vi "UHR-Fleezers Control (host) - 12.1_Jonathan.vi"() -> ()   [LabVIEW 2012] (continued)
                n283 = local read "Scan lines (y)"() -> (w520:u64)
                n284 = disable-structure shown="Disabled" {
                  frame Disabled {
                  }
                  frame Enabled {
                  }
                }
                n285 = local read "Actual MCL Inc (V)"() -> (w514:dbl)
                n286 = local read "Scan steps (MCL)"() -> (w519:u64)
                n287 = Divide "Y Pix/step"(x=w515, y=w520) -> (x/y=w527:dbl)
                n288 = Divide "Y V/pix"(x=w514, y=w527) -> (x/y=w526:dbl)
                n289 = Divide "Y half step offset"(x=w514, y=2.0) -> (x/y=w528:dbl)
                n290 = Divide "X pix/step"(x=w516, y=w519) -> (x/y=w525:dbl)
                n291 = Negate(x=w528) -> (-x=w529:dbl)
                n292 = local read "Initial Y"() -> (w535:dbl)
                n293 = Multiply(x=w517, y=w526) -> (x*y=w536:dbl)
                n294 = Divide "X half step offset"(x=w514, y=2.0) -> (x/y=w522:dbl)
                n295 = Divide "X V/pix"(x=w514, y=w525) -> (x/y=w524:dbl)
                n296 = Multiply(x=w514, y=w519) -> (x*y=w531:dbl)
                n297 = Compound Arithmetic op=ADD(w529, w536, w535) -> (w506:dbl)
                "Pointer Y (V)" <- w506
                n298 = Multiply(x=w524, y=w518) -> (x*y=w533:dbl)
                n299 = Negate(x=w522) -> (-x=w521:dbl)
                n300 = local read "Initial X"() -> (w534:dbl)
                n301 = Negate(x=w533) -> (-x=w532:dbl)
                n302 = Compound Arithmetic op=ADD(w521, w531, w534, w532) -> (w507:dbl)
                "Pointer X (V)" <- w507
                n303 = case shown="True" "Set High F Confocal Spot (X-Y)" {
                  tunnel: w507 -> [_ w537]
                  tunnel: w506 -> [_ w538]
                  frame False {
                  }
                  frame True {
                    "Confocal Y 2 (V)" <- w538
                    "Confocal X 2 (V)" <- w537
                  }
                }
                n304 = Or(x="Set X Only", y="Set Confocal Spot (X-Y)") -> (x .or. y?=w510:bool)
                n305 = Or(x="Set Confocal Spot (X-Y)", y="Set Y Only") -> (x .or. y?=w509:bool)
                n306 = case shown="True" w510 {
                  tunnel: w507 -> [_ w539]
                  frame False {
                  }
                  frame True {
                    n307 = property on="AO2" class="Slide (strict)"("Val(Sgnl)"=w539) -> ()  [unwired: 2 in, 2 out]
                    "Confocal X 1 (V)" <- w539
                  }
                }
                n308 = case shown="True" w509 {
                  tunnel: w506 -> [_ w540]
                  frame False {
                  }
                  frame True {
                    n309 = property on="AO1" class="Slide (strict)"("Val(Sgnl)"=w540) -> ()  [unwired: 2 in, 2 out]
                    "Confocal Y 1 (V)" <- w540
                  }
                }
                n310 = local write "Set High F Confocal Spot (X-Y)"(w505) -> ()
                n311 = local write "Set Confocal Spot (X-Y)"(w505) -> ()
                n312 = local write "Set X Only"(w505) -> ()
                n313 = local write "Set Y Only"(w505) -> ()
              }
            }
          }
          frame 3 {
            n314 = local read "BD 2 Frequency 1 (MHz)"() -> (w541:dbl)
            n315 = local read "BD 1 Frequency 1 (MHz)"() -> (w542:dbl)
            n316 = local write "Manipulating Trap"(TRUE ("Manipulating Trap")) -> ()
            n317 = local write "Coords"(T8 {"Horizontal"=0, "Vertical"=0} ("Coords")) -> ()
            n318 = while {
              tunnel: w547 -> [w552]
              tunnel: w545 -> [w551]
              tunnel: w543 -> [w550]
              tunnel: w542 -> [w549]
              tunnel: w541 -> [w548]
              stop <- w553 stop-if-true
              n319 = event shown="[0] \"Pane\": Mouse Move" {
                selector: _ -> [_ _]
                dyn-events: _ -> [_ _]
                timeout: _ -> [_ _]
                tunnel: ["Force Manip Abort" w617] -> w553
                tunnel: w552 -> [w560 _]
                tunnel: w551 -> [w558 _]
                tunnel: w550 -> [w557 _]
                tunnel: w549 -> [w556 _]
                tunnel: w548 -> [w555 _]
                event Mouse Move {
                  n320 = event-data() -> ("Time"=w561:u32, "Coords"=w562:T8)  [unwired: 3 out]
                  n321 = Less?(x=w561, y=w560) -> (x < y?=w559:bool)
                  n322 = case "Makes sure old motion events prior to mouse click aren't used" shown="False" w559 {
                    tunnel: w562 -> [w604 _]
                    tunnel: w558 -> [w605 _]
                    tunnel: w557 -> [w582 _]
                    tunnel: w556 -> [w578 _]
                    tunnel: w555 -> [w577 _]
                    frame False {
                      n323 = Subtract(x=w604, y=w605) -> (x-y=w603:T8)
                      "Coords" <- w603
                      n324 = local read "Y RF Frequency Limits (MHz)"() -> (w563:T17)
                      n325 = To Double Precision Float(number=w603) -> (double precision float=w602:cluster{"Horizontal":dbl, "Vertical":dbl})
                      n326 = Multiply(x=cluster{"Horizontal":dbl, "Vertical":dbl} {"Horizontal"=-1.0, "Vertical"=1.0}, y="Manipulation Scaling") -> (x*y=w598:cluster{"Horizontal":dbl, "Vertical":dbl})
                      n327 = local read "X RF Frequency Limits (MHz)"() -> (w564:T17)
                      n328 = Multiply(x=w602, y=w598) -> (x*y=w600:cluster{"Horizontal":dbl, "Vertical":dbl})
                      n329 = Unbundle By Name(w600) -> ("Horizontal"=w595:dbl, "Vertical"=w599:dbl)
                      n330 = Unbundle By Name(w563) -> ("Maximum"=w566:dbl, "Minimum"=w565:dbl)
                      n331 = Boolean To (0,1)(Boolean="Manip. X?") -> (0, 1=w593:i16)
                      n332 = Boolean To (0,1)(Boolean="Manip. Y?") -> (0, 1=w590:i16)
                      n333 = local read "BD 1 Frequency 2 (MHz)"() -> (w580:dbl)
                      n334 = Multiply(x=w599, y=w590) -> (x*y=w592:dbl)
                      n335 = Multiply(x=w593, y=w595) -> (x*y=w596:dbl)
                      n336 = local read "BD 2 Frequency 2 (MHz)"() -> (w579:dbl)
                      n337 = Unbundle By Name(w564) -> ("Maximum"=w568:dbl, "Minimum"=w567:dbl)
                      n338 = Add(x=w577, y=w592) -> (x+y=w570:dbl)
                      n339 = Add(x=w578, y=w596) -> (x+y=w572:dbl)
                      n340 = In Range and Coerce(upper limit=w568, x=w572, lower limit=w567) -> (coerced(x)=w571:dbl)  [unwired: 1 out]
                      n341 = In Range and Coerce(upper limit=w566, x=w570, lower limit=w565) -> (coerced(x)=w569:dbl)  [unwired: 1 out]
                      n342 = Subtract(x=w571, y=w580) -> (x-y=w589:dbl)
                      n343 = Subtract(x=w569, y=w579) -> (x-y=w588:dbl)
                      n344 = Square(x=w589) -> (x^2=w587:dbl)
                      n345 = Square(x=w588) -> (x^2=w586:dbl)
                      n346 = Add(x=w587, y=w586) -> (x+y=w585:dbl)
                      n347 = Square Root(x=w585) -> (sqrt(x)=w581:dbl)
                      n348 = In Range and Coerce(upper limit="Limit Max (MHz)", x=w581, lower limit="Limit Min (MHz)") -> (In Range?=w574:bool)  [unwired: 1 out]
                      n349 = Not(x="Limits Enable") -> (.not. x?=w573:bool)
                      n350 = Or(x=w574, y=w573) -> (x .or. y?=w575:bool)
                      n351 = case shown="True" w575 {
                        tunnel: w582 -> [_ w615]
                        tunnel: w581 -> [_ w606]
                        tunnel: w571 -> [_ w613]
                        tunnel: w580 -> [_ w612]
                        tunnel: w569 -> [_ w611]
                        tunnel: w579 -> [_ w610]
                        tunnel: w564 -> [_ w608]
                        tunnel: w563 -> [_ w607]
                        frame False {
                        }
                        frame True {
                          n352 = local read "BD 1 Frequency 3 (MHz)"() -> (w614:dbl)
                          n353 = local read "BD 2 Frequency 3 (MHz)"() -> (w609:dbl)
                          n354 = local write "Trap Delta (MHz)"(w606) -> ()
                          n355 = call "set RF board frequency - interlace.vi"("Board 2 Frequency Limits"=w607, "Board 1 Frequency Limits"=w608, "FPGA VI Reference In"=w615, "Board 2 Frequency 3 (MHz)"=w609, "Board 1 Frequency 3 (MHz)"=w614, "Board 2 Frequency 2 (MHz)"=w610, "Board 2 Frequency 1 (MHz)"=w611, "Board 1 Frequency 2 (MHz)"=w612, "Board 1 Frequency 1  (MHz)"=w613) -> ()  [unwired: 1 in, 2 out]
                          n356 = local write "BD 2 Frequency 1 (MHz)"(w611) -> ()
                          n357 = local write "BD 1 Frequency 1 (MHz)"(w613) -> ()
                        }
                      }
                    }
                    frame True {
                    }
                  }
                }
                event Mouse Up {
                  n358 = event-data() -> ("Button"=w616:u16)  [unwired: 8 out]
                  n359 = case shown="3" w616 {
                    tunnel: [FALSE TRUE] -> w617
                    frame 0, Default {
                    }
                    frame 3 {
                      n360 = local read "Trap Delta (MHz)"() -> (w619:dbl)
                      n361 = property on="Initial delta (MHz)" class="DigNum (strict)"("Val(Sgnl)"=w619) -> ()  [unwired: 2 in, 2 out]
                      n362 = local write "Manipulating Trap"(FALSE ("Manipulating Trap")) -> ()
                    }
                  }
                }
              }
            }
          }
        }
      }
      event Mouse Move {
        n363 = event-data() -> ()  [unwired: 6 out]
      }
    }
    n364 = local read "Stop All"() -> (w435:bool)
    n365 = node-c288() -> ()  [unwired: 2 out]
  }
  n366 = timed-loop "Run Scripts, including: stage motion" {
    tunnel: w91 -> [w628]
    tunnel: w90 -> [w629]
    tunnel: [w629] -> w89
    tunnel: [w628] -> w88
    timing: w86 -> [_]
    timing-out: [_] -> w85
    tunnel: w71 -> [w627]
    tunnel: w72 -> [w626]
    tunnel: w12 -> [w623]
    tunnel: w11 -> [w622]
    tunnel: w10 -> [w624]
    tunnel: w9 -> [w625]
    stop <- w630 stop-if-true
    n367 = node-c288() -> ()  [unwired: 1 in, 1 out]
    n368 = event shown="[3] \"Move Cap. 2 (ADig Top)\": Value Change" {
      selector: _ -> [_ _ _ _ _ _ _ _ _ _ _ _ _ _ _ _ _ _ _]
      dyn-events: _ -> [_ _ _ _ _ _ _ _ _ _ _ _ _ _ _ _ _ _ _]
      timeout: _ -> [_ _ _ _ _ _ _ _ _ _ _ _ _ _ _ _ _ _ _]
      tunnel: ["Set Position" "Move to Position" _ _ "Read Harvard" _ _ _ _ _ _ "Got ADig bead" "Force FB Data\nScript" _ "Got DNA bead" "Take Stepping Data" _ "Take Detection Laser\nImage" _] -> _
      tunnel: [_ _ _ _ _ _ _ _ _ _ _ _ _ _ _ _ _ _ w1247] -> w630
      tunnel: w628 -> [w648 w656 w669 w699 _ w744 w784 w865 w894 w1026 w1052 _ w1088 _ _ _ _ _ _]
      tunnel: w629 -> [w649 w657 w670 w700 _ w745 w785 w866 w895 w1027 w1053 _ w1089 _ _ _ _ _ _]
      tunnel: w627 -> [_ _ _ _ w729 _ _ _ _ _ _ _ _ _ _ _ _ _ _]
      tunnel: w626 -> [_ _ _ _ w728 _ _ _ _ _ _ _ _ _ _ _ _ _ _]
      tunnel: w625 -> [_ _ _ _ _ _ _ _ _ _ _ _ _ _ _ _ _ _ _]
      tunnel: w624 -> [_ _ _ _ _ _ _ _ _ _ _ _ _ _ _ _ _ _ _]
      tunnel: w623 -> [_ _ _ _ _ _ _ _ _ _ _ _ _ _ _ _ _ _ _]
      tunnel: w622 -> [_ _ _ _ _ _ _ _ _ _ _ _ _ _ _ _ _ _ _]
      event "Set Position", "Set Position 2", "Set Position 3", "Set Position 4", "Set Position 5", "Set Position 1": Value Change {
        n369 = event-data() -> ()  [unwired: 1 in, 5 out]
        n370 = Build Array("Set Position 1", "Set Position 2", "Set Position 3", "Set Position 4", "Set Position 5") -> (w647:bool[])
        n371 = Boolean Array To Number(Boolean array=w647) -> (number=w646:u32)
        n372 = Logarithm Base 2(1:w646) -> (0:w638:dbl)
        n373 = call "Read Stage Position.vi"("error in"=w648, "VISA resource name in"=w649) -> ("Current Position"=w653:cluster{dbl, dbl, dbl}, "error out"=w652:errorcluster)  [unwired: 2 out]
        n374 = Decrement(x="Position") -> (x-1=w636:dbl)
        n375 = Greater Or Equal?(x=w638, y=0.0) -> (x >= y?=w639:bool)
        n376 = Cluster To Array(cluster=w653) -> (array=w650:dbl[])
        n377 = local write "Stage Control Serial Error"(w652) -> ()
        n378 = Select(t=w638, s=w639, f=w636) -> (s? t:f=w635:dbl)
        n379 = Increment(x=w635) -> (x+1=w634:dbl)
        n380 = Build Array (concatenate)(w634, w650) -> (w633:dbl[])
        n381 = Replace Array Subset(array="Saved Stage Positions", new element=w633, index (row)=w635) -> (w651:dbl[][])  [unwired: 1 in]
        n382 = local write "Saved Stage Positions"(w651) -> ()
      }
      event "Move to Position": Value Change {
        n383 = event-data() -> ()  [unwired: 1 in, 5 out]
        n384 = flat-sequence {
          tunnel: w657 -> [w661]
          tunnel: w656 -> [w660]
          frame #0 {
            n385 = local read "Saved Stage Positions"() -> (w663:dbl[][])
            n386 = local read "Position"() -> (w662:dbl)
            n387 = local write "Stage Moving"(TRUE ("Stage Moving")) -> ()
            n388 = call "move to saved stage position.vi"("error in"=w660, "Stage VISA resource name in"=w661, "Position"=w662, "Saved Stage Positions"=w663) -> ("error out"=w659:errorcluster)  [unwired: 1 out]
            n389 = local write "Stage Control Serial Error"(w659) -> ()
          }
          frame #1 {
            n390 = call <vilib>:"Beep.vi"() -> ()  [unwired: 3 in, 9 out]
            n391 = local write "Stage Moving"(FALSE ("Stage Moving")) -> ()
          }
        }
      }
      event "Move Cap. 1 (DNA Bottom)": Value Change {
        n392 = event-data() -> ()  [unwired: 1 in, 5 out]
        n393 = local write "Move Cap. 1 (DNA Bottom)"(FALSE ("Move Cap. 1 (DNA Right)")) -> ()
        n394 = flat-sequence {
          tunnel: w669 -> [w672]
          tunnel: w670 -> [w673]
          tunnel: [w673] -> w667
          tunnel: [w672] -> w666
          tunnel: w667 -> [w675]
          tunnel: w666 -> [w674]
          frame #0 {
            n395 = property on="Sample Channel\nFlow" class="Bool (strict)"("Val(Sgnl)"="Cap 1 Samp Flow ON") -> ()  [unwired: 2 in, 2 out]
          }
          frame #1 {
            n396 = local read "Saved Stage Positions"() -> (w685:dbl[][])
            n397 = local write "Stage Moving"(TRUE ("Stage Moving")) -> ()
            n398 = Array Subset(array=w685, index (row)=0 ("index"), length (row)=1 ("length"), index (col)=1 ("index"), length (col)=3 ("length")) -> (w682:dbl[][])
            n399 = Reshape Array(w682, 3 ("dimension size")) -> (w680:dbl[])
            n400 = Array To Cluster(array=w680) -> (cluster=w679:cluster{"[0]":dbl, "[1]":dbl, "[2]":dbl})
            n401 = call "Set Stage Position.vi"("Position"=w679, "error in"=w674, "VISA resource name in"=w675) -> ("error out"=w678:errorcluster)  [unwired: 2 out]
            n402 = local write "Stage Control Serial Error"(w678) -> ()
          }
          frame #2 {
            n403 = local write "Stage Moving"(FALSE ("Stage Moving")) -> ()
            n404 = case shown="True" "Cap 1 Flow ON" {
              frame False {
              }
              frame True {
                n405 = property on="Inject Pump 1" class="Bool (strict)"("Val(Sgnl)"=TRUE ("Value (Signaling)")) -> ()  [unwired: 2 in, 2 out]
              }
            }
            n406 = call <vilib>:"Beep.vi"() -> ()  [unwired: 3 in, 9 out]
          }
          frame #3 {
            n407 = property on="Sample Channel\nFlow" class="Bool (strict)"("Val(Sgnl)"=FALSE ("Value (Signaling)")) -> ()  [unwired: 2 in, 2 out]
            n408 = local read "Cap. 2 BD T1?\n(ADig T1, DNA T2)"() -> (w692:bool)
            n409 = case shown="True" w692 {
              tunnel: "Cap 1 T ON" -> [w694 w695]
              frame False {
                n410 = property on="Trap 1 (ON/OFF)" class="Bool (strict)"("Val(Sgnl)"=w694) -> ()  [unwired: 2 in, 2 out]
              }
              frame True {
                n411 = property on="Trap 2 (ON/OFF)" class="Bool (strict)"("Val(Sgnl)"=w695) -> ()  [unwired: 2 in, 2 out]
              }
            }
            n412 = property on="Got DNA bead" class="Bool"("Key Focus"=TRUE) -> ()  [unwired: 2 in, 2 out]
          }
        }
      }
      event "Move Cap. 2 (ADig Top)": Value Change {
        n413 = event-data() -> ()  [unwired: 1 in, 5 out]
        n414 = local write "Move Cap. 2 (ADig Top)"(FALSE ("Move Cap. 2 (ADig Left)")) -> ()
        n415 = flat-sequence {
          tunnel: w699 -> [w702]
          tunnel: w700 -> [w703]
          tunnel: [w703] -> w697
          tunnel: [w702] -> w696
          tunnel: w697 -> [w706]
          tunnel: w696 -> [w705]
          frame #0 {
            n416 = property on="Sample Channel\nFlow" class="Bool (strict)"("Val(Sgnl)"="Cap 2 Samp Flow ON") -> ()  [unwired: 2 in, 2 out]
          }
          frame #1 {
            w704 = FALSE ("Value (Signaling)")
            n417 = local read "Saved Stage Positions"() -> (w716:dbl[][])
            n418 = local write "Stage Moving"(TRUE ("Stage Moving")) -> ()
            n419 = Array Subset(array=w716, index (row)=1 ("index"), length (row)=1 ("length"), index (col)=1 ("index"), length (col)=3 ("length")) -> (w713:dbl[][])
            n420 = Reshape Array(w713, 3 ("dimension size")) -> (w711:dbl[])
            n421 = property on="Trap 1 (ON/OFF)" class="Bool (strict)"("Val(Sgnl)"=w704) -> ()  [unwired: 2 in, 2 out]
            n422 = property on="Trap 1 (ON/OFF)" class="Bool (strict)"("Val(Sgnl)"=w704) -> ()  [unwired: 2 in, 2 out]
            n423 = Array To Cluster(array=w711) -> (cluster=w710:cluster{"[0]":dbl, "[1]":dbl, "[2]":dbl})
            n424 = call "Set Stage Position.vi"("Position"=w710, "error in"=w705, "VISA resource name in"=w706) -> ("error out"=w709:errorcluster)  [unwired: 2 out]
            n425 = local write "Stage Control Serial Error"(w709) -> ()
          }
          frame #2 {
            n426 = local write "Stage Moving"(FALSE ("Stage Moving")) -> ()
            n427 = call <vilib>:"Beep.vi"() -> ()  [unwired: 3 in, 9 out]
            n428 = case shown="True" "Cap 2 Flow ON" {
              frame False {
              }
              frame True {
                n429 = property on="Inject Pump 3" class="Bool (strict)"("Val(Sgnl)"=TRUE ("Value (Signaling)")) -> ()  [unwired: 2 in, 2 out]
              }
            }
          }
          frame #3 {
            n430 = property on="Sample Channel\nFlow" class="Bool (strict)"("Val(Sgnl)"=FALSE ("Value (Signaling)")) -> ()  [unwired: 2 in, 2 out]
            n431 = case shown="False" "Cap. 2 BD T1?\n(ADig T1, DNA T2)" {
              tunnel: "Cap 2 T ON" -> [w725 w726]
              frame False {
                n432 = property on="Trap 2 (ON/OFF)" class="Bool (strict)"("Val(Sgnl)"=w725) -> ()  [unwired: 2 in, 2 out]
              }
              frame True {
                n433 = property on="Trap 1 (ON/OFF)" class="Bool (strict)"("Val(Sgnl)"=w726) -> ()  [unwired: 2 in, 2 out]
              }
            }
            n434 = property on="Got ADig bead" class="Bool"("Key Focus"=TRUE) -> ()  [unwired: 2 in, 2 out]
          }
        }
      }
      event "Read Harvard": Value Change {
        n435 = event-data() -> ()  [unwired: 1 in, 5 out]
        n436 = Concatenate Strings("write buffer", "\r") -> (w731:string)
        n437 = VISA Write(VISA resource name=w729, write buffer=w731, error in (no error)=w728) -> (VISA resource name out=w740:refnum<visa-resource-name>, error out=w739:errorcluster)  [unwired: 1 out]
        n438 = stacked-sequence {
          tunnel: [w743] -> w738
          tunnel: w740 -> [w743]
          tunnel: w739 -> [w742]
          tunnel: [w742] -> w733
          frame #0 {
            n439 = Wait (ms)(milliseconds to wait=50) -> ()  [unwired: 1 out]
          }
        }
        n440 = property class="Instr"(reference=w738, error in=w733) -> (reference out=w737:refnum<visa-resource-name>, error out=w735:errorcluster, "Serial Settings:Number of Bytes at Serial Port"=w736:u32)
        "Serial Settings:Number of Bytes at Serial Port" <- w736
        n441 = VISA Read(VISA resource name=w737, byte count=w736, error in (no error)=w735) -> (read buffer=w734:string)  [unwired: 3 out]
        "read buffer" <- w734
        n442 = Fract/Exp String To Number(string=w734) -> ()  [unwired: 5 out]
      }
      event "+z", "-z": Value Change {
        n443 = event-data() -> ()  [unwired: 1 in, 5 out]
        n444 = flat-sequence {
          tunnel: w744 -> [w766]
          tunnel: w745 -> [w746]
          frame #0 {
            n445 = call "Read Stage Position.vi"("error in"=w766, "VISA resource name in"=w746) -> ("Current Position"=w751:cluster{dbl, dbl, dbl}, "error out"=w764:errorcluster, "VISA resource name out"=w765:refnum<visa-resource-name>)  [unwired: 1 out]
            n446 = local read "Saved Stage Positions"() -> (w775:dbl[][])
            n447 = Divide(x="z nudge increment (um)", y=1000.0) -> (x/y=w763:dbl)
            n448 = Boolean To (0,1)(Boolean="+z") -> (0, 1=w755:i16)
            n449 = Boolean To (0,1)(Boolean="-z") -> (0, 1=w756:i16)
            n450 = Array Subset(array=w775, index (row)=1 ("index"), length (row)=1 ("length"), index (col)=1 ("index"), length (col)=3 ("length")) -> (w772:dbl[][])
            n451 = Multiply(x=w755, y=w763) -> (x*y=w759:dbl)
            n452 = Multiply(x=w756, y=w763) -> (x*y=w757:dbl)
            n453 = Unbundle(w751) -> (w749:dbl, w748:dbl, w752:dbl)
            n454 = Negate(x=w757) -> (-x=w758:dbl)
            n455 = Reshape Array(w772, 3 ("dimension size")) -> (w770:dbl[])
            n456 = Add(x=w759, y=w758) -> (x+y=w760:dbl)
            n457 = Array To Cluster(array=w770) -> ()  [unwired: 1 out]
            n458 = Add(x=w760, y=w752) -> (x+y=w750:dbl)
            n459 = Bundle(cluster=w751, w749, w748, w750) -> (w747:cluster{dbl, dbl, dbl})
            n460 = call "Set Stage Position.vi"("Position"=w747, "error in"=w764, "VISA resource name in"=w765) -> ("error out"=w769:errorcluster)  [unwired: 2 out]
            n461 = local write "Stage Moving"(TRUE ("Stage Moving")) -> ()
            n462 = local write "Stage Control Serial Error"(w769) -> ()
          }
          frame #1 {
            n463 = local write "Stage Moving"(FALSE ("Stage Moving")) -> ()
            n464 = call <vilib>:"Beep.vi"() -> ()  [unwired: 3 in, 9 out]
          }
        }
      }
      event "Cal/Data Acq. Spot": Value Change {
        n465 = event-data() -> ()  [unwired: 1 in, 5 out]
        n466 = flat-sequence {
          tunnel: w784 -> [w788]
          tunnel: w785 -> [w789]
          tunnel: [w789] -> w781
          tunnel: [w788] -> w780
          tunnel: w781 -> [w794]
          tunnel: w780 -> [w793]
          tunnel: ["Cal @ (MHz)"] -> w778
          tunnel: [w798] -> w782
          tunnel: w778 -> [w798]
          tunnel: w782 -> [w807]
          tunnel: ["W/ Offset 1"] -> w779
          tunnel: w782 -> [w828]
          tunnel: w779 -> [w826]
          frame #0 {
            n467 = property on="Sample Channel\nFlow" class="Bool (strict)"("Val(Sgnl)"="Daq spot flow on") -> ()  [unwired: 2 in, 2 out]
            n468 = Wait (ms)(milliseconds to wait=u32 250) -> ()  [unwired: 1 out]
          }
          frame #1 {
            n469 = local read "Saved Stage Positions"() -> (w791:dbl[][])
            n470 = property on="Trap Delta (MHz)" class="DigNum (strict)"("Val(Sgnl)"="Cal @ (MHz)") -> ()  [unwired: 2 in, 2 out]
            n471 = local write "Stage Moving"(TRUE ("Stage Moving")) -> ()
            n472 = call "move to saved stage position.vi"("error in"=w793, "Stage VISA resource name in"=w794, "Position"="Cal Stage Position", "Saved Stage Positions"=w791) -> ("error out"=w792:errorcluster)  [unwired: 1 out]
            n473 = local write "Stage Control Serial Error"(w792) -> ()
          }
          frame #2 {
            n474 = local write "Stage Moving"(FALSE ("Stage Moving")) -> ()
            n475 = property on="Sample Channel\nFlow" class="Bool (strict)"("Val(Sgnl)"="Flow ON during cal?") -> ()  [unwired: 2 in, 2 out]
            n476 = call <vilib>:"Beep.vi"() -> ()  [unwired: 3 in, 9 out]
          }
          frame #3 {
            n477 = Wait (ms)(milliseconds to wait=u32 1000) -> ()  [unwired: 1 out]
          }
          frame #4 {
            n478 = property on="Save Calibration" class="Bool (strict)"("Val(Sgnl)"=TRUE ("Value (Signaling)")) -> ()  [unwired: 2 in, 2 out]
          }
          frame #5 {
            n479 = Wait (ms)(milliseconds to wait=u32 2000) -> ()  [unwired: 1 out]
          }
          frame #6 {
            # "Check to see if \nsaving done"
            n480 = while {
              stop <- w803 stop-if-true
              n481 = local read "Saving..."() -> (w804:bool)
              n482 = Wait (ms)(milliseconds to wait=u32 100) -> ()  [unwired: 1 out]
              n483 = Not(x=w804) -> (.not. x?=w803:bool)
            }
          }
          frame #7 {
            n484 = case shown="True" "W/ Offset 1" {
              tunnel: w807 -> [_ w808]
              frame False {
              }
              frame True {
                n485 = stacked-sequence {
                  tunnel: w808 -> [_ _ _ _ _ _ _ w825]
                  frame #0 {
                    n486 = property on="Trap Delta (MHz)" class="DigNum (strict)"("Val(Sgnl)"="Offset 1 Start (MHz)") -> ()  [unwired: 2 in, 2 out]
                    n487 = Replace Array Subset(array=u32[] [0] ("Index Values"), new element="Offset 1 Set", index=0) -> (w809:u32[])
                    n488 = property on="Saved AOD Raster Scan Parameter Sets" class="Arr (strict)"("Index Values"=w809) -> ()  [unwired: 2 in, 2 out]
                  }
                  frame #1 {
                    n489 = Wait (ms)(milliseconds to wait=u32 200) -> ()  [unwired: 1 out]
                  }
                  frame #2 {
                    n490 = property on="Load parameters" class="Bool (strict)"("Val(Sgnl)"=TRUE ("Value (Signaling)")) -> ()  [unwired: 2 in, 2 out]
                  }
                  frame #3 {
                    n491 = Wait (ms)(milliseconds to wait=u32 200) -> ()  [unwired: 1 out]
                  }
                  frame #4 {
                    n492 = property on="Trap Raster Scan" class="Bool (strict)"("Val(Sgnl)"=TRUE ("Value (Signaling)")) -> ()  [unwired: 2 in, 2 out]
                  }
                  frame #5 {
                    n493 = Wait (ms)(milliseconds to wait=u32 2000) -> ()  [unwired: 1 out]
                  }
                  frame #6 {
                    n494 = while {
                      stop <- w822 stop-if-true
                      n495 = local read "Raster Scanning..."() -> (w824:bool)
                      n496 = local read "Saving..."() -> (w820:bool)
                      n497 = Wait (ms)(milliseconds to wait=u32 100) -> ()  [unwired: 1 out]
                      n498 = Not(x=w820) -> (.not. x?=w819:bool)
                      n499 = Not(x=w824) -> (.not. x?=w821:bool)
                      n500 = And(x=w821, y=w819) -> (x .and. y?=w822:bool)
                    }
                  }
                  frame #7 {
                    n501 = property on="Trap Delta (MHz)" class="DigNum (strict)"("Val(Sgnl)"=w825) -> ()  [unwired: 2 in, 2 out]
                  }
                }
              }
            }
          }
          frame #8 {
            n502 = local read "Save ave N"() -> (w827:dbl)
            n503 = case shown="False" "W/ Offset 2" {
              tunnel: w828 -> [_ w835]
              tunnel: w827 -> [_ w834]
              tunnel: w826 -> [w830 _]
              frame False {
                n504 = case shown="False" w830 {
                  frame False {
                    n505 = Multiply(x="Cal read wait (s)", y=u32 1000 ("milliseconds to wait")) -> (x*y=w832:u32)
                    n506 = Wait (ms)(milliseconds to wait=w832) -> ()  [unwired: 1 out]
                  }
                  frame True {
                  }
                }
              }
              frame True {
                n507 = stacked-sequence {
                  tunnel: w835 -> [_ _ _ _ _ _ _ _ _ w856 _ _]
                  tunnel: w834 -> [_ _ _ _ _ _ _ _ _ w854 _ _]
                  frame #0 {
                    n508 = property on="Save ave N" class="DigNum (strict)"("Val(Sgnl)"=1.0 ("Value (Signaling)")) -> ()  [unwired: 2 in, 2 out]
                  }
                  frame #1 {
                    n509 = Wait (ms)(milliseconds to wait=u32 500) -> ()  [unwired: 1 out]
                  }
                  frame #2 {
                    n510 = property on="Trap Delta (MHz)" class="DigNum (strict)"("Val(Sgnl)"="Offset 2 Start (MHz)") -> ()  [unwired: 2 in, 2 out]
                    n511 = Replace Array Subset(array=u32[] [0] ("Index Values"), new element="Offset 2 Set", index=0) -> (w840:u32[])
                    n512 = property on="Saved AOD Raster Scan Parameter Sets" class="Arr (strict)"("Index Values"=w840) -> ()  [unwired: 2 in, 2 out]
                  }
                  frame #3 {
                    n513 = Wait (ms)(milliseconds to wait=u32 500) -> ()  [unwired: 1 out]
                  }
                  frame #4 {
                    n514 = property on="Load parameters" class="Bool (strict)"("Val(Sgnl)"=TRUE ("Value (Signaling)")) -> ()  [unwired: 2 in, 2 out]
                  }
                  frame #5 {
                    n515 = Wait (ms)(milliseconds to wait=u32 500) -> ()  [unwired: 1 out]
                  }
                  frame #6 {
                    n516 = property on="Trap Raster Scan" class="Bool (strict)"("Val(Sgnl)"=TRUE ("Value (Signaling)")) -> ()  [unwired: 2 in, 2 out]
                  }
                  frame #7 {
                    n517 = Wait (ms)(milliseconds to wait=u32 2000) -> ()  [unwired: 1 out]
                  }
                  frame #8 {
                    n518 = while {
                      stop <- w849 stop-if-true
                      n519 = local read "Raster Scanning..."() -> (w852:bool)
                      n520 = local read "Saving..."() -> (w850:bool)
                      n521 = Wait (ms)(milliseconds to wait=u32 100) -> ()  [unwired: 1 out]
                      n522 = Not(x=w850) -> (.not. x?=w848:bool)
                      n523 = Not(x=w852) -> (.not. x?=w851:bool)
                      n524 = And(x=w851, y=w848) -> (x .and. y?=w849:bool)
                    }
                  }
                  frame #9 {
                    n525 = property on="Trap Delta (MHz)" class="DigNum (strict)"("Val(Sgnl)"=w856) -> ()  [unwired: 2 in, 2 out]
                    n526 = property on="Saved AOD Raster Scan Parameter Sets" class="Arr (strict)"("Index Values"=u32[] [0]) -> ()  [unwired: 2 in, 2 out]
                    n527 = property on="Save ave N" class="DigNum (strict)"("Val(Sgnl)"=w854) -> ()  [unwired: 2 in, 2 out]
                  }
                  frame #10 {
                    n528 = Wait (ms)(milliseconds to wait=u32 500) -> ()  [unwired: 1 out]
                  }
                  frame #11 {
                    n529 = property on="Load parameters" class="Bool (strict)"("Val(Sgnl)"=TRUE ("Value (Signaling)")) -> ()  [unwired: 2 in, 2 out]
                  }
                }
              }
            }
          }
          frame #9 {
            n530 = property on="Read Cal" class="Bool (strict)"("Val(Sgnl)"=TRUE ("Value (Signaling)")) -> ()  [unwired: 2 in, 2 out]
          }
          frame #10 {
            n531 = Wait (ms)(milliseconds to wait=u32 1000) -> ()  [unwired: 1 out]
          }
          frame #11 {
            n532 = property on="Fish for Tether" class="Bool (strict)"("Val(Sgnl)"=TRUE ("Value (Signaling)")) -> ()  [unwired: 2 in, 2 out]
          }
        }
        n533 = local write "Cal/Data Acq. Spot"(FALSE ("Cal/Data Acq. Spot")) -> ()
      }
      event "Dump Beads": Value Change {
        n534 = event-data() -> ()  [unwired: 1 in, 5 out]
        n535 = flat-sequence {
          tunnel: ["Dump spot flow on?"] -> w862
          tunnel: [w873] -> w863
          tunnel: w862 -> [w873]
          tunnel: w866 -> [w878]
          tunnel: w865 -> [w877]
          tunnel: [w875] -> w864
          tunnel: w863 -> [w875]
          tunnel: w864 -> [w888]
          frame #0 {
            w867 = FALSE ("Value (Signaling)")
            n536 = local read "Saving..."() -> (w869:bool)
            n537 = local write "Dump Beads"(FALSE ("Dump Beads")) -> ()
            n538 = property on="Inject Pump 3" class="Bool (strict)"("Val(Sgnl)"=w867) -> ()  [unwired: 2 in, 2 out]
            n539 = property on="Inject Pump 1" class="Bool (strict)"("Val(Sgnl)"=w867) -> ()  [unwired: 2 in, 2 out]
            n540 = local write "Stop Saving"(w869) -> ()
          }
          frame #1 {
            w870 = FALSE ("Fl. Triggered...")
            n541 = case shown="True" "Dump spot flow on?" {
              frame False {
              }
              frame True {
                n542 = property on="Sample Channel\nFlow" class="Bool (strict)"("Val(Sgnl)"=TRUE ("Stage Moving")) -> ()  [unwired: 2 in, 2 out]
              }
            }
            n543 = local write "Fl. Triggered..."(w870) -> ()
            n544 = local write "Tether"(w870) -> ()
            n545 = property on="Green Laser ON/Interlacing" class="Bool (strict)"("Val(Sgnl)"=w870) -> ()  [unwired: 2 in, 2 out]
            n546 = property on="Trap Pos. FB ON" class="Bool (strict)"("Val(Sgnl)"=w870) -> ()  [unwired: 2 in, 2 out]
            n547 = property on="Trap Trig. Fl." class="Bool (strict)"("Val(Sgnl)"=w870) -> ()  [unwired: 2 in, 2 out]
            n548 = property on="Fl. Triggered..." class="Bool (strict)"("Val(Sgnl)"=w870) -> ()  [unwired: 2 in, 2 out]
            n549 = property on="Dip for Protein" class="Bool (strict)"("Val(Sgnl)"=w870) -> ()  [unwired: 2 in, 2 out]
            n550 = property on="Pause dwell" class="Bool (strict)"("Val(Sgnl)"=w870) -> ()  [unwired: 2 in, 2 out]
          }
          frame #2 {
            n551 = property on="Trap Pos. FB Offset Factor" class="DigNum (strict)"("Val(Sgnl)"=i64 0 ("Value (Signaling)")) -> ()  [unwired: 2 in, 2 out]
          }
          frame #3 {
            n552 = local read "Saved Stage Positions"() -> (w879:dbl[][])
            n553 = local write "Stage Moving"(TRUE ("Stage Moving")) -> ()
            n554 = Array Subset(array=w879, index (row)=3 ("index"), length (row)=1 ("length"), index (col)=1 ("index"), length (col)=3 ("length")) -> (w884:dbl[][])
            n555 = Reshape Array(w884, 3 ("dimension size")) -> (w882:dbl[])
            n556 = Array To Cluster(array=w882) -> (cluster=w881:cluster{"[0]":dbl, "[1]":dbl, "[2]":dbl})
            n557 = call "Set Stage Position.vi"("Position"=w881, "error in"=w877, "VISA resource name in"=w878) -> ()  [unwired: 3 out]
          }
          frame #4 {
            w889 = FALSE ("Value (Signaling)")
            n558 = case shown="True" w888 {
              frame False {
              }
              frame True {
                n559 = property on="Sample Channel\nFlow" class="Bool (strict)"("Val(Sgnl)"=FALSE ("Stage Moving")) -> ()  [unwired: 2 in, 2 out]
              }
            }
            n560 = property on="Trap 1 (ON/OFF)" class="Bool (strict)"("Val(Sgnl)"=w889) -> ()  [unwired: 2 in, 2 out]
            n561 = property on="Trap 2 (ON/OFF)" class="Bool (strict)"("Val(Sgnl)"=w889) -> ()  [unwired: 2 in, 2 out]
            n562 = call <vilib>:"Beep.vi"() -> ()  [unwired: 3 in, 9 out]
          }
          frame #5 {
            n563 = property on="Move Cap. 2 (ADig Top)" class="Bool (strict)"("Val(Sgnl)"=TRUE ("Value (Signaling)")) -> ()  [unwired: 2 in, 2 out]
            n564 = property on="Tab Control" class="TabCtl (strict)"("Val(Sgnl)"=T27."Status" ("Value (Signaling)")) -> ()  [unwired: 2 in, 2 out]
          }
        }
      }
      event "Dip for Protein": Value Change {
        n565 = event-data() -> ()  [unwired: 1 in, 5 out]
        n566 = case shown="True" "Dip for Protein" {
          tunnel: w895 -> [_ w897]
          tunnel: w894 -> [_ w896]
          frame False {
          }
          frame True {
            n567 = while {
              tunnel: w897 -> [w908]
              tunnel: w896 -> [w907]
              i -> [w902]
              stop <- w904 stop-if-true
              n568 = Increment(x=w902) -> (x+1=→"Dip #":i32)
              n569 = flat-sequence {
                tunnel: w907 -> [w919]
                tunnel: w908 -> [w920]
                tunnel: [w920] -> w912
                tunnel: [w919] -> w911
                tunnel: [w913] -> w898
                tunnel: [w925] -> w906
                tunnel: [w926] -> w905
                tunnel: w912 -> [w927]
                tunnel: w911 -> [w928]
                tunnel: [w923] -> w899
                tunnel: w898 -> [w923]
                tunnel: [w936] -> w910
                tunnel: w906 -> [w936]
                tunnel: [w935] -> w909
                tunnel: w905 -> [w935]
                tunnel: [w932] -> w903
                tunnel: [w931] -> w900
                tunnel: w899 -> [w931]
                tunnel: w909 -> [w956]
                tunnel: w910 -> [w957]
                tunnel: w903 -> [w958]
                tunnel: w900 -> [w955]
                tunnel: [w1014] -> w904
                frame #0 {
                  n570 = local read "Trap Pos. FB ON"() -> (w913:bool)
                  n571 = Compound Arithmetic op=AND("Flow ON\nduring dip?", "FB OFF when \nflow ON", w913) -> (w914:bool)
                  n572 = case shown="True" "Move trap \nbefore dip move?" {
                    frame False {
                    }
                    frame True {
                      n573 = property on="Trap Delta (MHz)" class="DigNum (strict)"("Val(Sgnl)"="Dipping Delta (MHz)") -> ()  [unwired: 2 in, 2 out]
                    }
                  }
                  n574 = property on="Green Laser ON/Interlacing" class="Bool (strict)"("Val(Sgnl)"="Green ON\nbefore dip?") -> ()  [unwired: 2 in, 2 out]
                  n575 = property on="Sample Channel\nFlow" class="Bool (strict)"("Val(Sgnl)"="Flow ON\nduring dip?") -> ()  [unwired: 2 in, 2 out]
                  n576 = case shown="True" w914 {
                    frame False {
                    }
                    frame True {
                      n577 = property on="Trap Pos. FB ON" class="Bool (strict)"("Val(Sgnl)"=FALSE ("Value (Signaling)")) -> ()  [unwired: 2 in, 2 out]
                    }
                  }
                }
                frame #1 {
                  n578 = local read "Saved Stage Positions"() -> (w930:dbl[][])
                  n579 = local write "Cancel dwell"(FALSE ("Cancel dwell")) -> ()
                  n580 = call "move to saved stage position.vi"("error in"=w928, "Stage VISA resource name in"=w927, "Position"="Dip Stage \nPosition", "Saved Stage Positions"=w930) -> ("VISA resource name out"=w925:refnum<visa-resource-name>, "error out"=w926:errorcluster)
                }
                frame #2 {
                  n581 = node-c288() -> (w934:T22)  [unwired: 4 in]
                  n582 = timed-loop {
                    timing: w934 -> [_]
                    timing-out: [_] -> w933
                    tunnel: [w940] -> w932
                    i -> [w937]
                    stop <- w941 stop-if-true
                    n583 = node-c288() -> ()  [unwired: 1 in, 1 out]
                    n584 = Greater Or Equal?(x=w937, y="Dip Duration (s)") -> (x >= y?=w949:bool)
                    n585 = local read "Dip for Protein"() -> (w942:bool)
                    n586 = local read "Dump Beads"() -> (w939:bool)
                    n587 = local read "Cancel dwell"() -> (w948:bool)
                    n588 = local read "Pause dwell"() -> (w945:bool)
                    n589 = Not(x=w942) -> (.not. x?=w947:bool)
                    n590 = Compound Arithmetic op=OR(w948, w949, w947) -> (w946:bool)
                    n591 = Select(t=FALSE, s=w945, f=w946) -> (s? t:f=w943:bool)
                    n592 = Not(x=w939) -> (.not. x?=w938:bool)
                    n593 = node-c288() -> ()  [unwired: 1 in, 1 out]
                    n594 = And(x=w942, y=w938) -> (x .and. y?=w940:bool)
                    n595 = Or(x=w943, y=w939) -> (x .or. y?=w941:bool)
                    "Dip Time (s)" <- w937
                  }
                  n596 = node-c288(w933) -> ()  [unwired: 1 out]
                }
                frame #3 {
                  n597 = case shown="True" w958 {
                    tunnel: w957 -> [_ w963]
                    tunnel: w956 -> [_ w962]
                    tunnel: w955 -> [_ w959]
                    frame False {
                    }
                    frame True {
                      n598 = flat-sequence {
                        tunnel: w962 -> [w967]
                        tunnel: w963 -> [w968]
                        tunnel: [w968] -> w961
                        tunnel: [w967] -> w960
                        tunnel: w959 -> [w964]
                        tunnel: w961 -> [w978]
                        tunnel: w960 -> [w977]
                        tunnel: w959 -> [w986]
                        frame #0 {
                          n599 = local read "Sample Channel\nFlow"() -> (w966:bool)
                          n600 = case shown="True" w966 {
                            tunnel: "Flow ON \nduring return\nfrom dip?" -> [w969 w972]
                            tunnel: w964 -> [_ w971]
                            frame False {
                              n601 = case shown="True" w969 {
                                frame False {
                                }
                                frame True {
                                n602 = property on="Sample Channel\nFlow" class="Bool (strict)"("Val(Sgnl)"=TRUE ("Value (Signaling)")) -> ()  [unwired: 2 in, 2 out]
                                }
                              }
                            }
                            frame True {
                              n603 = case shown="False" w972 {
                                tunnel: w971 -> [w973 _]
                                frame False {
                                n604 = property on="Trap Pos. FB ON" class="Bool (strict)"("Val(Sgnl)"=w973) -> ()  [unwired: 2 in, 2 out]
                                n605 = property on="Sample Channel\nFlow" class="Bool (strict)"("Val(Sgnl)"=FALSE ("Value (Signaling)")) -> ()  [unwired: 2 in, 2 out]
                                }
                                frame True {
                                }
                              }
                            }
                          }
                        }
                        frame #1 {
                          # "For turning on green laser before stage reaches lower spot"
                          n606 = case shown="True" "Green ON\nafter start\nreturn?" {
                            frame False {
                            }
                            frame True {
                              n607 = flat-sequence {
                                frame #0 {
                                n608 = Multiply(x="Green delay after \nstart return (s)", y=1000.0) -> (x*y=w983:dbl)
                                n609 = Wait (ms)(milliseconds to wait=w983) -> ()  [unwired: 1 out]
                                }
                                frame #1 {
                                n610 = property on="Green Laser ON/Interlacing" class="Bool (strict)"("Val(Sgnl)"=TRUE ("Value (Signaling)")) -> ()  [unwired: 2 in, 2 out]
                                }
                              }
                            }
                          }
                          n611 = local read "Saved Stage Positions"() -> (w981:dbl[][])
                          n612 = local write "Cancel dwell"(FALSE ("Cancel dwell")) -> ()
                          n613 = call "move to saved stage position.vi"("error in"=w977, "Stage VISA resource name in"=w978, "Position"="Return Stage \nPosition", "Saved Stage Positions"=w981) -> ("error out"=w979:errorcluster)  [unwired: 1 out]
                          n614 = local write "Stage Control Serial Error"(w979) -> ()
                        }
                        frame #2 {
                          n615 = property on="Trap Pos. FB ON" class="Bool (strict)"("Val(Sgnl)"=w986) -> ()  [unwired: 2 in, 2 out]
                          n616 = case shown="True" "Green ON \nafter return?" {
                            frame False {
                            }
                            frame True {
                              n617 = property on="Green Laser ON/Interlacing" class="Bool (strict)"("Val(Sgnl)"=TRUE ("Value (Signaling)")) -> ()  [unwired: 2 in, 2 out]
                            }
                          }
                          n618 = case shown="True" "Move trap after return?" {
                            frame False {
                            }
                            frame True {
                              n619 = property on="Trap Delta (MHz)" class="DigNum (strict)"("Val(Sgnl)"="Dip Trap Delta 2 (MHz)") -> ()  [unwired: 2 in, 2 out]
                            }
                          }
                          n620 = case shown="True" "Save data after return?" {
                            frame False {
                            }
                            frame True {
                              n621 = property on="Start Saving" class="Bool (strict)"("Val(Sgnl)"=TRUE ("Value (Signaling)")) -> ()  [unwired: 2 in, 2 out]
                            }
                          }
                          n622 = property on="Sample Channel\nFlow" class="Bool (strict)"("Val(Sgnl)"="Flow ON\nduring daq?") -> ()  [unwired: 2 in, 2 out]
                        }
                        frame #3 {
                          n623 = node-c288() -> (w995:T22)  [unwired: 4 in]
                          n624 = timed-loop {
                            timing: w995 -> [_]
                            timing-out: [_] -> w994
                            i -> [w996]
                            stop <- w998 stop-if-true
                            n625 = node-c288() -> ()  [unwired: 1 in, 1 out]
                            n626 = local read "Dump Beads"() -> (w997:bool)
                            n627 = Greater Or Equal?(x=w996, y="Dwell Duration (s)") -> (x >= y?=w1003:bool)
                            n628 = local read "Dip for Protein"() -> (w1000:bool)
                            n629 = Not(x=w1000) -> (.not. x?=w999:bool)
                            n630 = Compound Arithmetic op=OR(w1003, "Cancel dwell", w999) -> (w1002:bool)
                            n631 = node-c288() -> ()  [unwired: 1 in, 1 out]
                            n632 = Select(t=FALSE, s="Pause dwell", f=w1002) -> (s? t:f=w1005:bool)
                            n633 = Or(x=w1005, y=w997) -> (x .or. y?=w998:bool)
                            "Dwell Time (s)" <- w996
                          }
                          n634 = node-c288(w994) -> ()  [unwired: 1 out]
                        }
                      }
                    }
                  }
                }
                frame #4 {
                  n635 = local read "Dip for Protein"() -> (w1015:bool)
                  n636 = local read "Dump Beads"() -> (w1012:bool)
                  n637 = local write "Cancel dwell"(FALSE ("Cancel dwell")) -> ()
                  n638 = Not(x=w1015) -> (.not. x?=w1016:bool)
                  n639 = Not(x="Cont. Repeat Dipping?") -> (.not. x?=w1018:bool)
                  n640 = Compound Arithmetic op=OR(w1016, w1018, w1012) -> (w1014:bool)
                }
              }
            }
          }
        }
      }
      event "Profile": Value Change {
        n641 = event-data() -> ()  [unwired: 1 in, 5 out]
        n642 = flat-sequence {
          tunnel: w1027 -> [w1030]
          tunnel: w1026 -> [w1038]
          tunnel: [w1032] -> w1025
          tunnel: [w1031] -> w1024
          tunnel: [w1029] -> w1022
          tunnel: [w1028] -> w1019
          tunnel: w1025 -> [w1045]
          tunnel: w1024 -> [w1044]
          tunnel: [w1042] -> w1023
          tunnel: w1022 -> [w1043]
          tunnel: [w1041] -> w1021
          tunnel: [w1040] -> w1020
          tunnel: w1019 -> [w1040]
          tunnel: w1023 -> [w1049]
          tunnel: w1021 -> [w1048]
          tunnel: w1020 -> [w1047]
          frame #0 {
            n643 = call "Read Stage Position.vi"("error in"=w1038, "VISA resource name in"=w1030) -> ("Current Position"=w1028:cluster{dbl, dbl, dbl}, "error out"=w1031:errorcluster, "VISA resource name out"=w1029:refnum<visa-resource-name>)  [unwired: 1 out]
            "Current Position" <- w1028
            n644 = local write "Stage Control Serial Error"(w1031) -> ()
            n645 = Unbundle(w1028) -> (w1035:dbl, w1037:dbl, w1033:dbl)
            n646 = Add(x=w1037, y="Y change (mm)") -> (x+y=w1034:dbl)
            n647 = Bundle(w1035, w1034, w1033) -> (w1032:cluster{dbl, dbl, dbl})  [unwired: 1 in]
          }
          frame #1 {
            # "move to new position and start saving"
            n648 = local write "Stage Moving"(TRUE ("Stage Moving")) -> ()
            n649 = local write "Start Saving"(TRUE ("Start Saving")) -> ()
            n650 = call "Set Stage Position.vi"("Position"=w1045, "error in"=w1044, "VISA resource name in"=w1043) -> ("error out"=w1041:errorcluster, "VISA resource name out"=w1042:refnum<visa-resource-name>)  [unwired: 1 out]
          }
          frame #2 {
            # "go back to start"
            n651 = call "Set Stage Position.vi"("Position"=w1047, "error in"=w1048, "VISA resource name in"=w1049) -> ()  [unwired: 3 out]
          }
          frame #3 {
            # "stop saving"
            n652 = local write "Stop Saving"(TRUE ("Stop Saving")) -> ()
            n653 = local write "Stage Moving"(FALSE ("Stage Moving")) -> ()
          }
        }
      }
      event "Move to Position 1", "Move to Position 2", "Move to Position 3", "Move to Position 4", "Move to Position 5", "Lower Ch. Cap.": Value Change {
        n654 = event-data() -> ()  [unwired: 1 in, 5 out]
        n655 = Or(x="Move to Position 5", y="Lower Ch. Cap.") -> (x .or. y?=w1055:bool)
        n656 = Build Array("Move to Position 1", "Move to Position 2", "Move to Position 3", "Move to Position 4", w1055) -> (w1058:bool[])
        n657 = Boolean Array To Number(Boolean array=w1058) -> (number=w1057:u32)
        n658 = Logarithm Base 2(1:w1057) -> (0:w1056:dbl)
        n659 = flat-sequence {
          tunnel: w1056 -> [w1067]
          tunnel: w1053 -> [w1065]
          tunnel: w1052 -> [w1064]
          frame #0 {
            n660 = local read "Saved Stage Positions"() -> (w1075:dbl[][])
            n661 = Array Subset(array=w1075, index (row)=w1067, length (row)=1 ("length"), index (col)=1 ("index"), length (col)=3 ("length")) -> (w1072:dbl[][])
            n662 = Reshape Array(w1072, 3 ("dimension size")) -> (w1070:dbl[])
            n663 = Array To Cluster(array=w1070) -> (cluster=w1069:cluster{"[0]":dbl, "[1]":dbl, "[2]":dbl})
            n664 = call "Set Stage Position.vi"("Position"=w1069, "error in"=w1064, "VISA resource name in"=w1065) -> ("error out"=w1068:errorcluster)  [unwired: 2 out]
            n665 = local write "Stage Moving"(TRUE ("Stage Moving")) -> ()
            n666 = local write "Stage Control Serial Error"(w1068) -> ()
          }
          frame #1 {
            n667 = local write "Stage Moving"(FALSE ("Stage Moving")) -> ()
            n668 = call <vilib>:"Beep.vi"() -> ()  [unwired: 3 in, 9 out]
          }
        }
      }
      event "Got ADig bead": Value Change {
        n669 = event-data() -> ()  [unwired: 1 in, 5 out]
        n670 = flat-sequence {
          frame #0 {
            n671 = local read "Cap 1 Samp Flow ON"() -> (w1079:bool)
            n672 = case shown="True" w1079 {
              frame False {
              }
              frame True {
                n673 = property on="Sample Channel\nFlow" class="Bool (strict)"("Val(Sgnl)"=TRUE ("Value (Signaling)")) -> ()  [unwired: 2 in, 2 out]
              }
            }
          }
          frame #1 {
            n674 = property on="Inject Pump 3" class="Bool (strict)"("Val(Sgnl)"=FALSE ("Value (Signaling)")) -> ()  [unwired: 2 in, 2 out]
          }
          frame #2 {
            n675 = property on="Move Cap. 1 (DNA Bottom)" class="Bool (strict)"("Val(Sgnl)"=TRUE ("Value (Signaling)")) -> ()  [unwired: 2 in, 2 out]
          }
        }
      }
      event "Force FB Data\nScript": Value Change {
        n676 = event-data() -> ()  [unwired: 1 in, 5 out]
        n677 = flat-sequence {
          tunnel: w1088 -> [w1092]
          tunnel: w1089 -> [w1093]
          tunnel: [w1093] -> w1084
          tunnel: [w1092] -> w1083
          tunnel: w1084 -> [w1096]
          tunnel: w1083 -> [w1095]
          tunnel: ["Trap Trig Fl."] -> w1085
